vi "StartModsICDAS.vi"(6 "Visualization VI Paths":path[](array[path]), 7 "ShowPanel? (f)":bool=TRUE, 8 "Error Array In":errorcluster[](array[cluster]), 9 "INI File Paths":path[](array[path]), 10 "Module List":string[](array[string]), 11 "Test.lvclass":refnum<class "Test.lvclass">) -> (0 "Error Array Out":errorcluster[](array[cluster]), 2 "Event Array":variant[](array[variant]), 3 "Test.lvclass":refnum<class "Test.lvclass">)   [LabVIEW 2018, in "Test.lvclass"]
doc: "Instantiates a module based on the module list."
uses:
  Test.lvclass
  Test.lvclass/Test.ctl
  <userlib>/NIST/ModuleAdminLib/ModuleAdmin/ModuleAdmin.lvclass/ModuleAdmin.ctl
  <userlib>/NIST/ModuleAdminLib/CloneRegistration/CloneRegistration.lvclass
  <userlib>/NIST/ModuleAdminLib/ModuleAdmin/Accessors/Read CloneRegRef.vi
  Accessors/Read ModuleList.vi
  Accessors/Read ModuleIDs.vi
  Accessors/Read CloneReg.vi
  Accessors/Write ModuleList.vi
  Accessors/Write ModuleIDs.vi
  Accessors/Write CloneReg.vi
  Sync/SyncModule/Main.vi
  FGen/FgenModule/Main.vi
  Analysis/AnalysisModule/Main.vi
  <vilib>/Utility/error.llb/Error Cluster From Error Code.vi
  <vilib>/ErrorRing/Error Ring.xnode
  <userlib>/NIST/ModuleAdminLib/ModuleAdmin/ModuleAdmin.lvclass
  <userlib>/NIST/NISTErrorLib/NISTErrorLib.lvlib
  Sync/SyncModule/SyncModule.lvlib
  Digitizer/DigitizerModule/DigitizerModule.lvlib
  FGen/FgenModule/FgenModule.lvlib
  Analysis/AnalysisModule/AnalysisModule.lvlib
  Sensor/SensorModule/SensorModule.lvlib
  Scope/ScopeModule/ScopeModule.lvlib
  AcPwr/AcPwrModule/AcPwrModule.lvlib
  AcPwr/AcPwrShared/AcPwrShared.lvlib
  Scope/ScopeShared/ScopeShared.lvlib
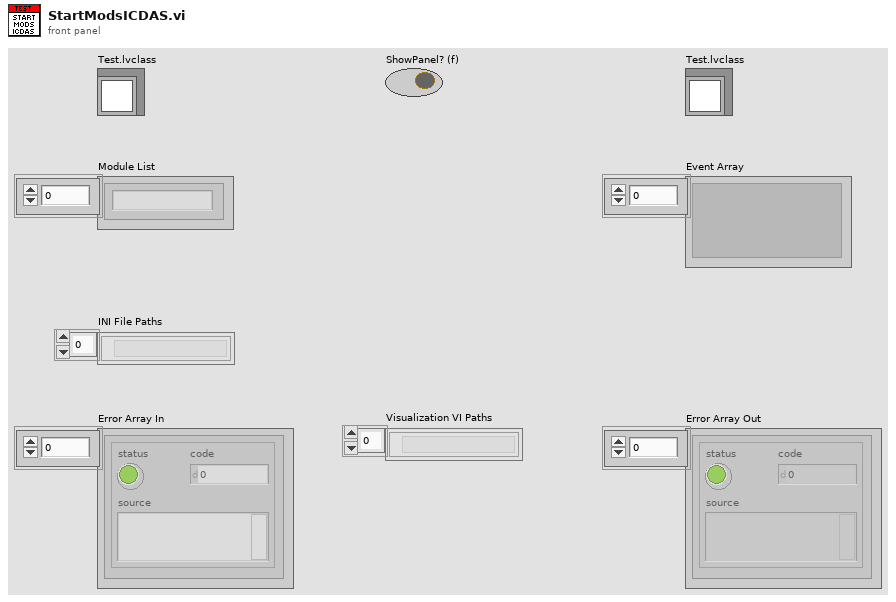
[diagram p1: front panel]
types:
  T1 = typedef "SyncModule.lvlib/clBroadcastEvents.ctl" = cluster{"DidInit":refnum<user-event>, "StatusUpdate":refnum<user-event>, "ErrorReport":refnum<user-event>, "DidStop":refnum<user-event>, "PathToINI":refnum<user-event>, "TriggerTime":refnum<user-event>, "LockStatus":refnum<user-event>, "Info":refnum<user-event>, "ClockProperties":refnum<user-event>}
  T2 = typedef "FgenModule.lvlib/clBroadcastEvents.ctl" = cluster{"DidInit":refnum<user-event>, "StatusUpdate":refnum<user-event>, "ErrorReport":refnum<user-event>, "DidStop":refnum<user-event>, "PathToINI":refnum<user-event>, "Channels":refnum<user-event>, "Function":refnum<user-event>, "Waveforms":refnum<user-event>, "Triggers":refnum<user-event>, "FunctionParams":refnum<user-event>, "FunctionArbs":refnum<user-event>, "FunctionSampleRate":refnum<user-event>}
  T3 = typedef "DigitizerShared.lvlib/clBroadcastEvents.ctl" = cluster{"DidInit":refnum<user-event>, "StatusUpdate":refnum<user-event>, "ErrorReport":refnum<user-event>, "DidStop":refnum<user-event>, "PathToINI":refnum<user-event>, "Channels":refnum<user-event>, "Acq":refnum<user-event>, "Trigger":refnum<user-event>, "Waveforms":refnum<user-event>}
  T4 = typedef "ScopeShared.lvlib/clBroadcastEvents.ctl" = cluster{"DidInit":refnum<user-event>, "StatusUpdate":refnum<user-event>, "ErrorReport":refnum<user-event>, "DidStop":refnum<user-event>, "PathToINI":refnum<user-event>, "Handle":refnum<user-event>, "Model":refnum<user-event>, "Channels":refnum<user-event>, "Acquisition":refnum<user-event>, "Trigger":refnum<user-event>, "ExtAcquisition":refnum<user-event>, "Waveform":refnum<user-event>}
  T5 = typedef "SensorShared.lvlib/clBroadcastEvents.ctl" = cluster{"DidInit":refnum<user-event>, "StatusUpdate":refnum<user-event>, "ErrorReport":refnum<user-event>, "DidStop":refnum<user-event>, "PathToINI":refnum<user-event>, "SensorReport":refnum<user-event>, "SensorConfig":refnum<user-event>}
  T6 = typedef "AnalysisModule.lvlib/clBroadcastEvents.ctl" = cluster{"DidInit":refnum<user-event>, "StatusUpdate":refnum<user-event>, "ErrorReport":refnum<user-event>, "DidStop":refnum<user-event>, "PathToINI":refnum<user-event>, "Config":refnum<user-event>, "ResultReport":refnum<user-event>, "FunctionClass":refnum<user-event>, "State":refnum<user-event>, "FunctionParams":refnum<user-event>, "Duration":refnum<user-event>}
  T7 = typedef "AcPwrShared.lvlib/AcPwrBroadcastEvents.ctl" = cluster{"DidInit":refnum<user-event>, "StatusUpdate":refnum<user-event>, "ErrorReport":refnum<user-event>, "DidStop":refnum<user-event>, "PathToINI":refnum<user-event>, "Measurements":refnum<user-event>, "LoadConfigFile":refnum<user-event>, "GetSettings":refnum<user-event>, "SetSettings":refnum<user-event>, "GetType&ID":refnum<user-event>, "GotSettings":refnum<user-event>}
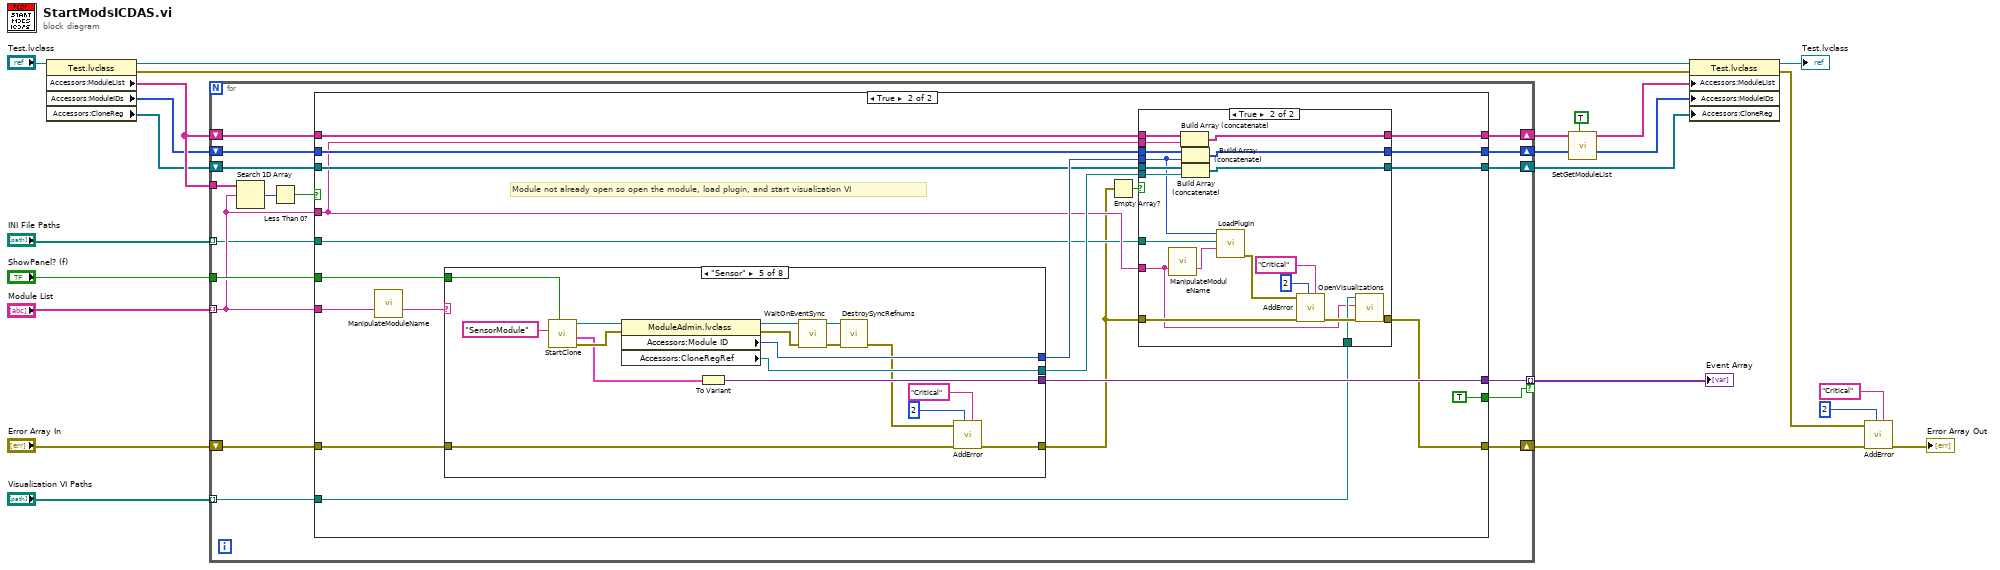
[diagram p0: block diagram]
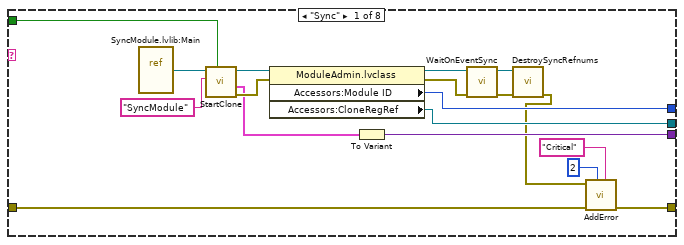
[diagram p4: hidden frame]
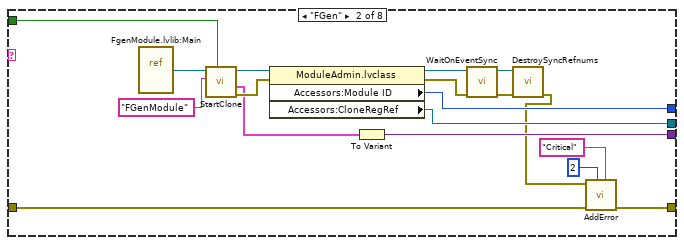
[diagram p5: hidden frame]
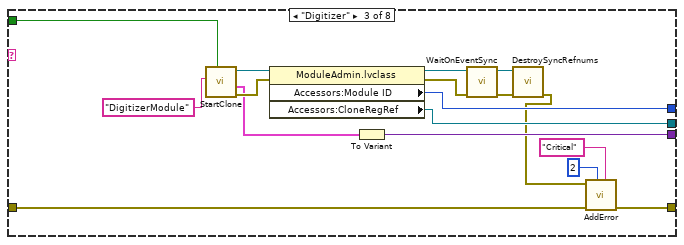
[diagram p6: hidden frame]
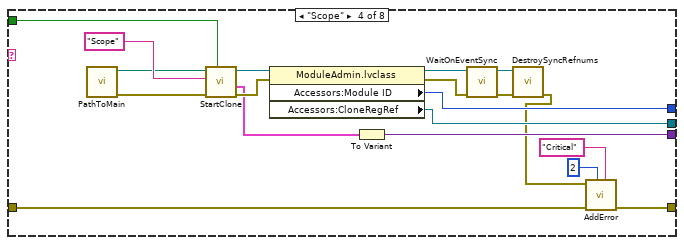
[diagram p7: hidden frame]
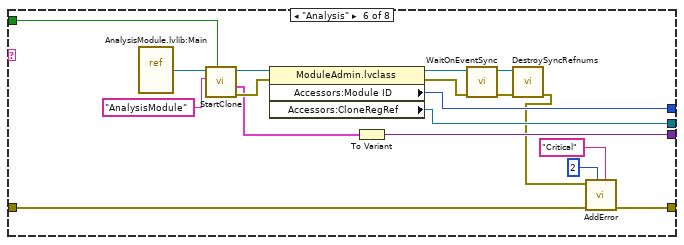
[diagram p8: hidden frame]
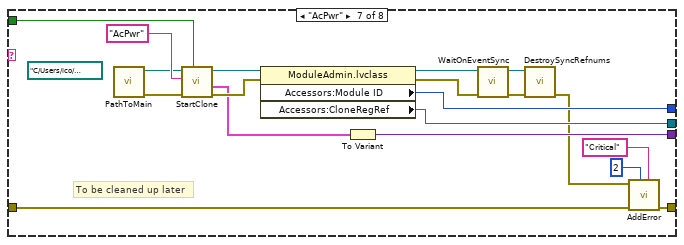
[diagram p9: hidden frame]
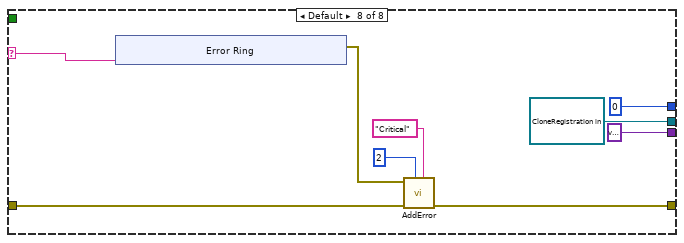
[diagram p10: hidden frame]
diagram:
  n1 = property class="Test.lvclass"(reference="Test.lvclass") -> (reference out=w12:refnum<class "Test.lvclass">, error out=w11:errorcluster, "Accessors:ModuleList"=w10:string[], "Accessors:ModuleIDs"=w9:i32[], "Accessors:CloneReg"=w8:refnum<data-value>[])  [unwired: 1 in]
  n2 = for {
    tunnel: "ShowPanel? (f)" -> [w40]
    tunnel: "Module List" -> [w32] mode=indexing
    tunnel: [w38] -> w16 mode=indexing if=w26
    shift-right: [w39] -> w19
    shift-left: "Error Array In" -> [w37]
    tunnel: w10 -> [w36]
    shift-right: [w27] -> w7
    shift-left: w10 -> [w33]
    shift-right: [w29] -> w6
    shift-left: w9 -> [w31]
    shift-right: [w28] -> w5
    shift-left: w8 -> [w30]
    tunnel: "INI File Paths" -> [w25] mode=indexing
    tunnel: "Visualization VI Paths" -> [w24] mode=indexing
    n3 = Search 1D Array(1D array=w36, element=w32) -> (index of element=w35:i32)  [unwired: 1 in]
    n4 = Less Than 0?(x=w35) -> (x < 0?=w34:bool)
    n5 = case shown="True" w34 {
      tunnel: w40 -> [_ w64]
      tunnel: [w41 w45] -> w39
      tunnel: w32 -> [_ w61]
      tunnel: [_ w63] -> w38
      tunnel: w37 -> [w41 w62]
      tunnel: w33 -> [w44 w59]
      tunnel: w32 -> [_ w49]
      tunnel: w31 -> [w43 w58]
      tunnel: w30 -> [w42 w56]
      tunnel: [w43 w54] -> w29
      tunnel: [w42 w53] -> w28
      tunnel: [w44 w52] -> w27
      tunnel: [_ TRUE] -> w26
      tunnel: w25 -> [_ w48]
      tunnel: w24 -> [_ w47]
      frame False {
        # "module open and plugin already loaded"
      }
      frame True {
        # "Module not already open so open the module, load plugin, and start visualization VI"
        n6 = call "ManipulateModuleName.vi"("ModuleListSingleEntry"=w61) -> ("BeforeMatch:ModuleListSingleEntry"=w60:string)  [unwired: 9 in, 5 out]
        n7 = case shown="\"Sensor\"" w60 {
          selector: w60 -> [_ _ _ _ _ _ _ w222]
          tunnel: w62 -> [w90 w108 w126 w145 w162 w179 w199 w221]
          tunnel: [w93 w111 w129 w148 w165 w182 w202 w217] -> w46
          tunnel: [w94 w112 w130 w149 w166 w183 w203 variant ("Variant")] -> w63
          tunnel: [w96 w114 w132 w151 w168 w185 w205 refnum<data-value> refnum ("Accessors:CloneRegRef")] -> w55
          tunnel: [w95 w113 w131 w150 w167 w184 w204 0 ("Accessors:Module ID")] -> w57
          tunnel: w64 -> [w88 w106 w124 w143 w160 w177 w197 _]
          frame "Sync" {
            n8 = vi-ref "SyncModule.lvlib:Main.vi"() -> (w105:refnum<vi>)
            n9 = call "StartClone.vi"("ShowPanel? (f)"=w88, "ModuleName"="SyncModule", "VI Refnum"=w105) -> ("error out"=w98:errorcluster, "SyncBroadcastEvents"=w97:T1, "ModuleAdmin"=w103:refnum<class "ModuleAdmin.lvclass">)  [unwired: 6 in]
            n10 = property class="ModuleAdmin.lvclass"(reference=w103, error in=w98) -> (reference out=w101:refnum<class "ModuleAdmin.lvclass">, error out=w102:errorcluster, "Accessors:Module ID"=w95:i32, "Accessors:CloneRegRef"=w96:refnum<data-value>)
            n11 = To Variant(anything=w97) -> (Variant=w94:variant)
            n12 = call <userlib>:"WaitOnEventSync.vi"("error in (no error)"=w102, "ModuleAdmin"=w101) -> ("error out"=w100:errorcluster, "ModuleAdmin"=w99:refnum<class "ModuleAdmin.lvclass">)  [unwired: 8 in]
            n13 = call <userlib>:"DestroySyncRefnums.vi"("error in (no error)"=w100, "ModuleAdmin"=w99) -> ("error out"=w89:errorcluster)  [unwired: 9 in]
            n14 = call <userlib>:"AddError.vi"("Severity"="Critical", "Priority"=u8 2, "ErrorArray In"=w90, "error in (no error)"=w89) -> ("ErrorArray Out"=w93:errorcluster[])  [unwired: 6 in, 1 out]
          }
          frame "FGen" {
            n15 = vi-ref "FgenModule.lvlib:Main.vi"() -> (w123:refnum<vi>)
            n16 = call "StartClone.vi"("ShowPanel? (f)"=w106, "ModuleName"="FGenModule", "VI Refnum"=w123) -> ("error out"=w116:errorcluster, "clBroadcastEvents"=w115:T2, "ModuleAdmin"=w121:refnum<class "ModuleAdmin.lvclass">)  [unwired: 6 in]
            n17 = property class="ModuleAdmin.lvclass"(reference=w121, error in=w116) -> (reference out=w119:refnum<class "ModuleAdmin.lvclass">, error out=w120:errorcluster, "Accessors:Module ID"=w113:i32, "Accessors:CloneRegRef"=w114:refnum<data-value>)
            n18 = To Variant(anything=w115) -> (Variant=w112:variant)
            n19 = call <userlib>:"WaitOnEventSync.vi"("error in (no error)"=w120, "ModuleAdmin"=w119) -> ("error out"=w118:errorcluster, "ModuleAdmin"=w117:refnum<class "ModuleAdmin.lvclass">)  [unwired: 8 in]
            n20 = call <userlib>:"DestroySyncRefnums.vi"("error in (no error)"=w118, "ModuleAdmin"=w117) -> ("error out"=w107:errorcluster)  [unwired: 9 in]
            n21 = call <userlib>:"AddError.vi"("Severity"="Critical", "Priority"=u8 2, "ErrorArray In"=w108, "error in (no error)"=w107) -> ("ErrorArray Out"=w111:errorcluster[])  [unwired: 6 in, 1 out]
          }
          frame "Digitizer" {
            n22 = call "StartClone.vi"("ShowPanel? (f)"=w124, "ModuleName"="DigitizerModule") -> ("error out"=w134:errorcluster, "clBroadcastEvents"=w133:T3, "ModuleAdmin"=w139:refnum<class "ModuleAdmin.lvclass">)  [unwired: 7 in]
            n23 = property class="ModuleAdmin.lvclass"(reference=w139, error in=w134) -> (reference out=w137:refnum<class "ModuleAdmin.lvclass">, error out=w138:errorcluster, "Accessors:Module ID"=w131:i32, "Accessors:CloneRegRef"=w132:refnum<data-value>)
            n24 = To Variant(anything=w133) -> (Variant=w130:variant)
            n25 = call <userlib>:"WaitOnEventSync.vi"("error in (no error)"=w138, "ModuleAdmin"=w137) -> ("error out"=w136:errorcluster, "ModuleAdmin"=w135:refnum<class "ModuleAdmin.lvclass">)  [unwired: 8 in]
            n26 = call <userlib>:"DestroySyncRefnums.vi"("error in (no error)"=w136, "ModuleAdmin"=w135) -> ("error out"=w125:errorcluster)  [unwired: 9 in]
            n27 = call <userlib>:"AddError.vi"("Severity"="Critical", "Priority"=u8 2, "ErrorArray In"=w126, "error in (no error)"=w125) -> ("ErrorArray Out"=w129:errorcluster[])  [unwired: 6 in, 1 out]
          }
          frame "Scope" {
            n28 = call "PathToMain.vi"() -> ("Error Out"=w142:errorcluster, "PathToMain"=w141:path)  [unwired: 10 in]
            n29 = call "StartClone.vi"("ShowPanel? (f)"=w143, "error in (no error)"=w142, "ModuleName"="Scope", "vi path"=w141) -> ("error out"=w153:errorcluster, "clBroadcastEvents"=w152:T4, "ModuleAdmin"=w158:refnum<class "ModuleAdmin.lvclass">)  [unwired: 5 in]
            n30 = property class="ModuleAdmin.lvclass"(reference=w158, error in=w153) -> (reference out=w156:refnum<class "ModuleAdmin.lvclass">, error out=w157:errorcluster, "Accessors:Module ID"=w150:i32, "Accessors:CloneRegRef"=w151:refnum<data-value>)
            n31 = To Variant(anything=w152) -> (Variant=w149:variant)
            n32 = call <userlib>:"WaitOnEventSync.vi"("error in (no error)"=w157, "ModuleAdmin"=w156) -> ("error out"=w155:errorcluster, "ModuleAdmin"=w154:refnum<class "ModuleAdmin.lvclass">)  [unwired: 8 in]
            n33 = call <userlib>:"DestroySyncRefnums.vi"("error in (no error)"=w155, "ModuleAdmin"=w154) -> ("error out"=w144:errorcluster)  [unwired: 9 in]
            n34 = call <userlib>:"AddError.vi"("Severity"="Critical", "Priority"=u8 2, "ErrorArray In"=w145, "error in (no error)"=w144) -> ("ErrorArray Out"=w148:errorcluster[])  [unwired: 6 in, 1 out]
          }
          frame "Sensor" {
            n35 = call "StartClone.vi"("ShowPanel? (f)"=w160, "ModuleName"="SensorModule") -> ("error out"=w170:errorcluster, "clBroadcastEvents"=w169:T5, "ModuleAdmin"=w175:refnum<class "ModuleAdmin.lvclass">)  [unwired: 7 in]
            n36 = property class="ModuleAdmin.lvclass"(reference=w175, error in=w170) -> (reference out=w173:refnum<class "ModuleAdmin.lvclass">, error out=w174:errorcluster, "Accessors:Module ID"=w167:i32, "Accessors:CloneRegRef"=w168:refnum<data-value>)
            n37 = To Variant(anything=w169) -> (Variant=w166:variant)
            n38 = call <userlib>:"WaitOnEventSync.vi"("error in (no error)"=w174, "ModuleAdmin"=w173) -> ("error out"=w172:errorcluster, "ModuleAdmin"=w171:refnum<class "ModuleAdmin.lvclass">)  [unwired: 8 in]
            n39 = call <userlib>:"DestroySyncRefnums.vi"("error in (no error)"=w172, "ModuleAdmin"=w171) -> ("error out"=w161:errorcluster)  [unwired: 9 in]
            n40 = call <userlib>:"AddError.vi"("Severity"="Critical", "Priority"=u8 2, "ErrorArray In"=w162, "error in (no error)"=w161) -> ("ErrorArray Out"=w165:errorcluster[])  [unwired: 6 in, 1 out]
          }
          frame "Analysis" {
            n41 = vi-ref "AnalysisModule.lvlib:Main.vi"() -> (w194:refnum<vi>)
            n42 = call "StartClone.vi"("ShowPanel? (f)"=w177, "ModuleName"="AnalysisModule", "VI Refnum"=w194) -> ("error out"=w187:errorcluster, "AnalysisBroadcastEvents"=w186:T6, "ModuleAdmin"=w192:refnum<class "ModuleAdmin.lvclass">)  [unwired: 6 in]
            n43 = property class="ModuleAdmin.lvclass"(reference=w192, error in=w187) -> (reference out=w190:refnum<class "ModuleAdmin.lvclass">, error out=w191:errorcluster, "Accessors:Module ID"=w184:i32, "Accessors:CloneRegRef"=w185:refnum<data-value>)
            n44 = To Variant(anything=w186) -> (Variant=w183:variant)
            n45 = call <userlib>:"WaitOnEventSync.vi"("error in (no error)"=w191, "ModuleAdmin"=w190) -> ("error out"=w189:errorcluster, "ModuleAdmin"=w188:refnum<class "ModuleAdmin.lvclass">)  [unwired: 8 in]
            n46 = call <userlib>:"DestroySyncRefnums.vi"("error in (no error)"=w189, "ModuleAdmin"=w188) -> ("error out"=w178:errorcluster)  [unwired: 9 in]
            n47 = call <userlib>:"AddError.vi"("Severity"="Critical", "Priority"=u8 2, "ErrorArray In"=w179, "error in (no error)"=w178) -> ("ErrorArray Out"=w182:errorcluster[])  [unwired: 6 in, 1 out]
          }
          frame "AcPwr" {
            (unwired) path "C:/Users/ico/Documents/Projects/NistPluggableModules/AcPwr/AcPwrPlugins/Common/Main.vi" ("vi path")
            # "To be cleaned up later"
            n48 = call "PathToMain.vi"() -> ("Error Out"=w196:errorcluster, "PathToMain"=w195:path)  [unwired: 10 in]
            n49 = call "StartClone.vi"("ShowPanel? (f)"=w197, "error in (no error)"=w196, "ModuleName"="AcPwr", "vi path"=w195) -> ("error out"=w207:errorcluster, "clAcPwrEvents"=w206:T7, "ModuleAdmin"=w212:refnum<class "ModuleAdmin.lvclass">)  [unwired: 5 in]
            n50 = property class="ModuleAdmin.lvclass"(reference=w212, error in=w207) -> (reference out=w210:refnum<class "ModuleAdmin.lvclass">, error out=w211:errorcluster, "Accessors:Module ID"=w204:i32, "Accessors:CloneRegRef"=w205:refnum<data-value>)
            n51 = To Variant(anything=w206) -> (Variant=w203:variant)
            n52 = call <userlib>:"WaitOnEventSync.vi"("error in (no error)"=w211, "ModuleAdmin"=w210) -> ("error out"=w209:errorcluster, "ModuleAdmin"=w208:refnum<class "ModuleAdmin.lvclass">)  [unwired: 8 in]
            n53 = call <userlib>:"DestroySyncRefnums.vi"("error in (no error)"=w209, "ModuleAdmin"=w208) -> ("error out"=w198:errorcluster)  [unwired: 9 in]
            n54 = call <userlib>:"AddError.vi"("Severity"="Critical", "Priority"=u8 2, "ErrorArray In"=w199, "error in (no error)"=w198) -> ("ErrorArray Out"=w202:errorcluster[])  [unwired: 6 in, 1 out]
          }
          frame Default {
            n55 = xnode "Error Ring"("parameter 0"=w222) -> ("error out"=w220:errorcluster)
            n56 = call <userlib>:"AddError.vi"("Severity"="Critical", "Priority"=u8 2, "ErrorArray In"=w221, "error in (no error)"=w220) -> ("ErrorArray Out"=w217:errorcluster[])  [unwired: 6 in, 1 out]
          }
        }
        n57 = Empty Array?(array=w46) -> (empty?=w51:bool)
        n58 = case shown="True" w51 {
          tunnel: w59 -> [w68 w87]
          tunnel: w49 -> [_ w86]
          tunnel: w58 -> [w66 w85]
          tunnel: w57 -> [_ w79]
          tunnel: w56 -> [w67 w84]
          tunnel: w55 -> [_ w83]
          tunnel: [w66 w82] -> w54
          tunnel: [w67 w81] -> w53
          tunnel: [w68 w69] -> w52
          tunnel: w49 -> [_ w70]
          tunnel: w48 -> [_ w78]
          tunnel: w46 -> [w65 w74]
          tunnel: w47 -> [_ w72]
          tunnel: [w65 w71] -> w45
          frame False {
          }
          frame True {
            n59 = call "ManipulateModuleName.vi"("ModuleListSingleEntry"=w70) -> ("BeforeMatch:ModuleListSingleEntry"=w80:string)  [unwired: 9 in, 5 out]
            n60 = Build Array (concatenate)(w87, w86) -> (w69:string[])
            n61 = Build Array (concatenate)(w85, w79) -> (w82:i32[])
            n62 = Build Array (concatenate)(w84, w83) -> (w81:refnum<data-value>[])
            n63 = call "LoadPlugin.vi"("Module Name"=w80, "INI File Path"=w78, "Module ID"=w79) -> ("error out"=w75:errorcluster)  [unwired: 5 in, 3 out]
            n64 = call <userlib>:"AddError.vi"("Severity"="Critical", "Priority"=u8 2, "ErrorArray In"=w74, "error in (no error)"=w75) -> ("ErrorArray Out"=w73:errorcluster[])  [unwired: 6 in, 1 out]
            n65 = call "OpenVisualizations.vi"("ErrorArray in"=w73, "Module Name"=w70, "Visualization VI Path"=w72) -> ("ErrorArray out"=w71:errorcluster[])  [unwired: 8 in]
          }
        }
      }
    }
  }
  "Event Array" <- w16
  n66 = call "SetGetModuleList.vi"("Set? (F)"=TRUE, "ModuleList"=w7) -> ("ModuleList"=w2:string[])  [unwired: 9 in]
  n67 = property class="Test.lvclass"(reference=w12, error in=w11, "Accessors:ModuleList"=w2, "Accessors:ModuleIDs"=w6, "Accessors:CloneReg"=w5) -> (reference out=→"Test.lvclass":refnum<class "Test.lvclass">, error out=w18:errorcluster)
  n68 = call <userlib>:"AddError.vi"("Severity"="Critical", "Priority"=u8 2, "ErrorArray In"=w19, "error in (no error)"=w18) -> ("ErrorArray Out"=→"Error Array Out":errorcluster[])  [unwired: 6 in, 1 out]
